vi "Interpolate Data with Fracational Ratio.vi"(10 "Ratio":dbl, 11 "Orgin":dbl[](array[numeric])) -> (3 "new array":dbl[](array[numeric]))   [LabVIEW 2017]
doc: "Resamples Orgin by the given Ratio using linear interpolation, so the output array length is the input length multiplied by Ratio."
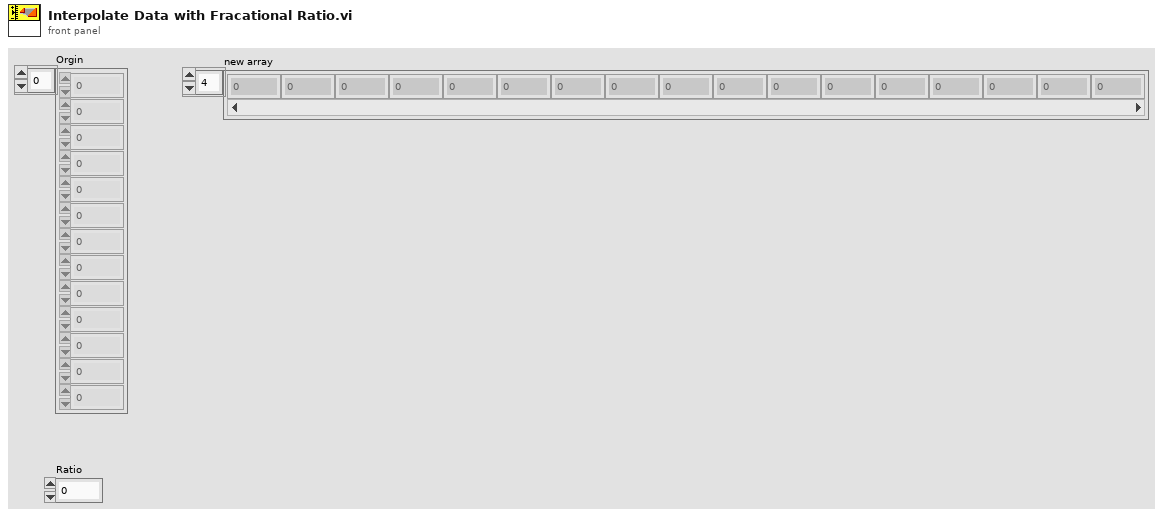
[diagram p1: front panel]
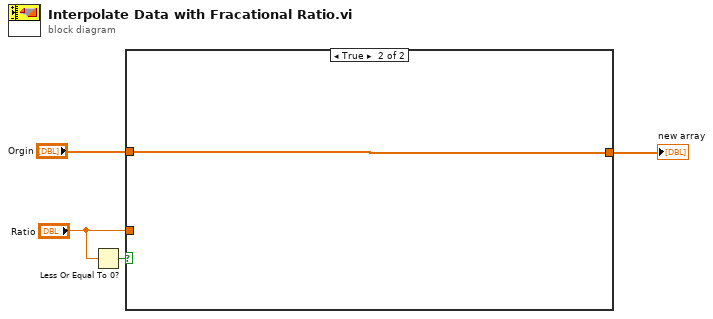
[diagram p0: block diagram]
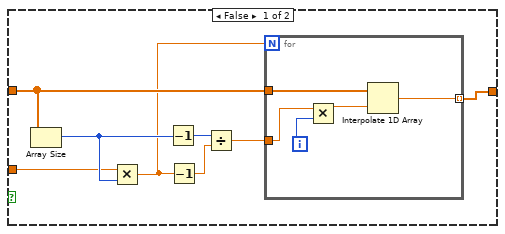
[diagram p2: hidden frame]
diagram:
  n1 = Less Or Equal To 0?(x="Ratio") -> (x <= 0?=w1:bool)
  n2 = case shown="True" w1 {
    tunnel: "Orgin" -> [w9 w18]
    tunnel: [w6 w18] -> w3
    tunnel: "Ratio" -> [w5 _]
    frame False {
      n3 = Array Size(array=w9) -> (size(s)=w8:i32)
      n4 = Multiply(x=w5, y=w8) -> (x*y=w7:dbl)
      n5 = Decrement(x=w8) -> (x-1=w11:i32)
      n6 = Decrement(x=w7) -> (x-1=w10:dbl)
      n7 = Divide(x=w11, y=w10) -> (x/y=w12:dbl)
      n8 = for {
        N: w7 -> [_]
        tunnel: w9 -> [w17]
        tunnel: w12 -> [w14]
        tunnel: [w15] -> w6 mode=indexing
        i -> [w16]
        n9 = Multiply(x=w14, y=w16) -> (x*y=w13:dbl)
        n10 = Interpolate 1D Array(1:w13, 2:w17) -> (0:w15:dbl)
      }
    }
    frame True {
    }
  }
  "new array" <- w3
